vi "Open HW References.vi"(11 "Module Azimuth Config Data":T2) -> (0 "Error Out":errorcluster, 1 "CANcoder Ref Out":T1, 2 "Module Drive Ref Out":T4, 3 "Module Steer Ref Out":T4)   [LabVIEW 2023, in "2024 AdvSwerve_ACT.lvlib"]
uses:
  2024 AdvSwerve_ACT.lvlib
  <vilib>/Rock Robotics/WPI/MotorControl/WPI_MotorControlDeviceRef.ctl
  <vilib>/Rock Robotics/WPI/MotorControl/WPI_MotorControlType.ctl
  <vilib>/Rock Robotics/SystemInterfaces/DIO/FPGA_DIOPWMChannel.ctl
  <vilib>/Rock Robotics/WPI/PWM/WPI_PWMDeadband.ctl
  <vilib>/Rock Robotics/SystemInterfaces/DIO/FPGA_DIOChannel.ctl
  Cluster_Config Specific Data.ctl
  Shared Code/TypeDefs/ENUM_Module Position.ctl
  <vilib>/Rock Robotics/WPI/ThirdParty/REV Robotics/REVLib/Typedef/Spark MAX Motor Type.ctl
  <vilib>/Rock Robotics/WPI/ThirdParty/Phoenix-LabVIEW/CANCoder/Controls/CTRE_Phoenix_CANcoder_DeviceRef.ctl
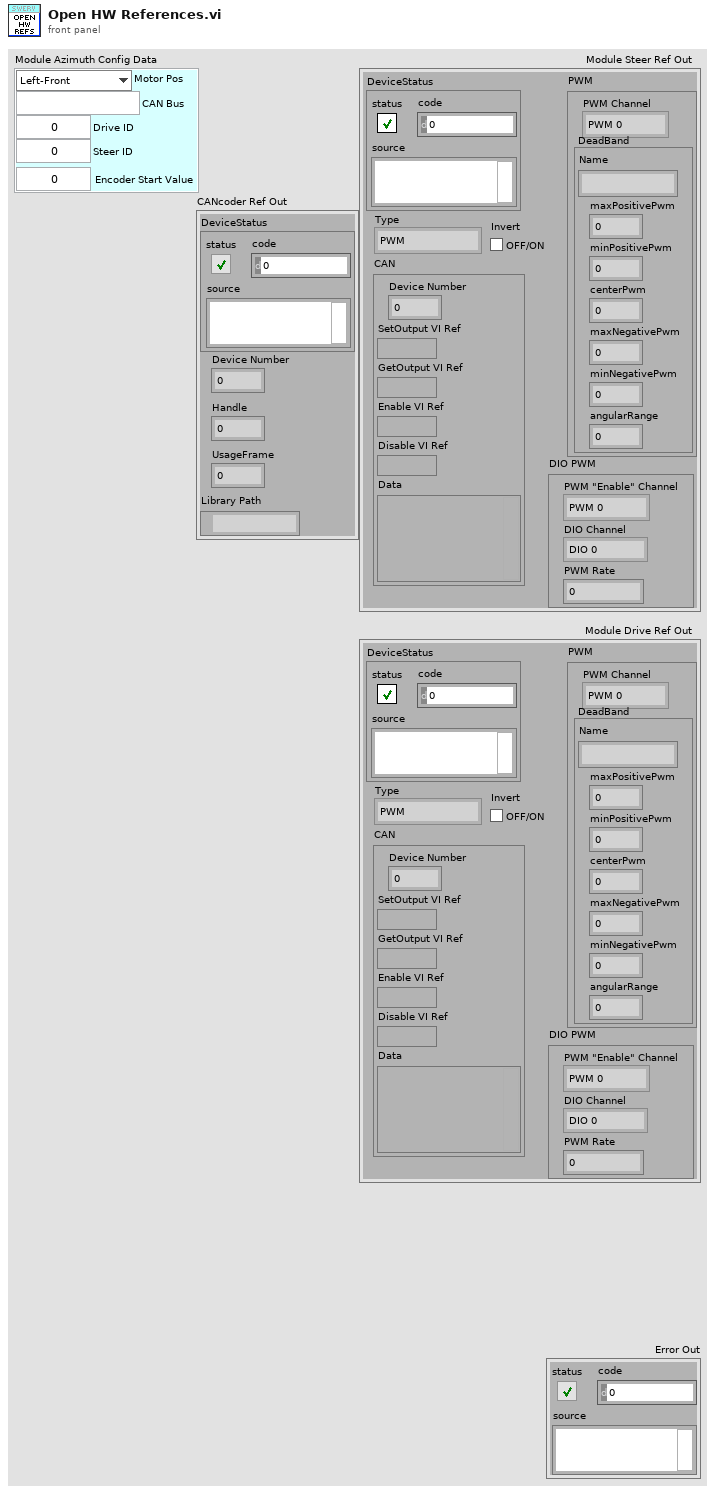
[diagram p1: front panel]
types:
  T1 = typedef "CTRE_Phoenix_CANcoder_DeviceRef.ctl" = cluster{"DeviceStatus":errorcluster, "Device Number":u8, "Handle":u64, "UsageFrame":u32, "Library Path":path}
  T2 = typedef "2024 AdvSwerve_ACT.lvlib/Cluster_Config Specific Data.ctl" = cluster{"Motor Pos":T3, "CAN Bus":string, "Drive ID":u8, "Steer ID":u8, "Encoder Start Value":dbl}
  T3 = typedef "ENUM_Module Position.ctl" = enum16{"Left-Front", "Right-Front", "Left-Back", "Right-Back"}
  T4 = typedef "WPI_MotorControlDeviceRef.ctl" = cluster{"DeviceStatus":errorcluster, "Type":T5, "PWM":cluster{"PWM Channel":T6, "DeadBand":T7}, "CAN":cluster{"Device Number":u8, "SetOutput VI Ref":variant, "GetOutput VI Ref":variant, "Enable VI Ref":variant, "Disable VI Ref":variant, "Data":variant}, "Invert":bool, "DIO PWM":cluster{"PWM \"Enable\" Channel":T6, "DIOChannel":T8, "PWM Rate":dbl}}
  T5 = typedef "WPI_MotorControlType.ctl" = enum16{"PWM", "CAN", "DIO PWM"}
  T6 = typedef "FPGA_DIOPWMChannel.ctl" = enum8{"PWM 0", "PWM 1", "PWM 2", "PWM 3", "PWM 4", "PWM 5", "PWM 6", "PWM 7", "PWM 8", "PWM 9", "PWM MXP 0", "PWM MXP 1", "PWM MXP 2", "PWM MXP 3", "PWM MXP 4", "PWM MXP 5", "PWM MXP 6", "PWM MXP 7", "PWM MXP 8", "PWM MXP 9", "Invalid"}
  T7 = typedef "WPI_PWMDeadband.ctl" = cluster{"Name":string, "maxPositivePwm":i32, "minPositivePwm":i32, "centerPwm":i32, "maxNegativePwm":i32, "minNegativePwm":i32, "angularRange":u16}
  T8 = typedef "FPGA_DIOChannel.ctl" = enum8{"DIO 0", "DIO 1", "DIO 2", "DIO 3", "DIO 4", "DIO 5", "DIO 6", "DIO 7", "DIO 8", "DIO 9", "DIO MXP 0", "DIO MXP 1", "DIO MXP 2", "DIO MXP 3", "DIO MXP 4", "DIO MXP 5", "DIO MXP 6", "DIO MXP 7", "DIO MXP 8", "DIO MXP 9", "DIO MXP 10", "DIO MXP 11", "DIO MXP 12", "DIO MXP 13", "DIO MXP 14", "DIO MXP 15", "SPI Port CS1", "SPI Port CS2", "SPI Port CS3", "SPI Port MISO", "SPI Port MOSI", "Invalid"}
  T9 = typedef "Spark MAX Motor Type.ctl" = enum16{"Brushed", "Brushless"}
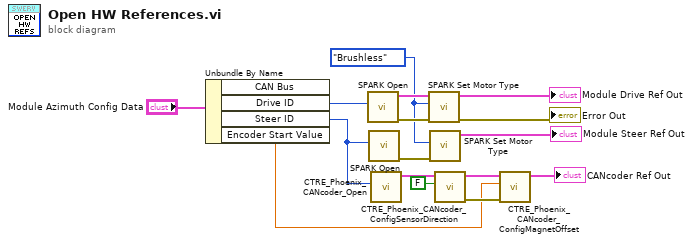
[diagram p0: block diagram]
diagram:
  w1 = Spark_MAX_Motor_Type."Brushless" ("Motor Type")
  n1 = Unbundle By Name("Module Azimuth Config Data") -> ("Drive ID"=w16:u8, "Steer ID"=w8:u8, "Encoder Start Value"=w2:dbl)  [unwired: 1 out]
  n2 = call <vilib>:"SPARK Open.vi"("Device Number"=w16) -> ("error out"=w11:errorcluster, "MotorControlDeviceRef"=w13:T4)  [unwired: 9 in]
  n3 = call <vilib>:"SPARK Open.vi"("Device Number"=w8) -> ("error out"=w10:errorcluster)  [unwired: 9 in, 1 out]
  n4 = call <vilib>:"CTRE_Phoenix_CANcoder_Open.vi"("Device Number"=w8) -> ("CTRE_CANcoder_DeviceRef"=w7:T1)  [unwired: 9 in, 1 out]
  n5 = call <vilib>:"SPARK Set Motor Type.vi"("error in (no error)"=w11, "Motor Type"=w1, "MotorControlDevRef"=w13) -> ("error out"=→"Error Out":errorcluster, "MotorControlDeviceRef"=→"Module Drive Ref Out":T4)  [unwired: 7 in]
  n6 = call <vilib>:"SPARK Set Motor Type.vi"("error in (no error)"=w10, "Motor Type"=w1) -> ("MotorControlDeviceRef"=→"Module Steer Ref Out":T4)  [unwired: 8 in, 1 out]
  n7 = call <vilib>:"CTRE_Phoenix_CANcoder_ConfigSensorDirection.vi"("Sensor Direction"=FALSE, "CTRE_CANcoder_DeviceRef"=w7) -> ("error out"=w5:errorcluster, "CTRE_CANcoder_DeviceRef"=w4:T1)  [unwired: 8 in]
  n8 = call <vilib>:"CTRE_Phoenix_CANcoder_ConfigMagnetOffset.vi"("error in"=w5, "Magnet Offset (Degrees)"=w2, "CTRE_CANcoder_DeviceRef"=w4) -> ("CTRE_CANcoder_DeviceRef"=→"CANcoder Ref Out":T1)  [unwired: 7 in, 1 out]
